vi "Fetch.vi"(6 "Prune Branches?":bool, 8 "error in (no error)":errorcluster, 10 "Name/Remote URL":string, 11 "Git Implementation in":refnum<class "Git Implementation.lvclass">) -> (0 "error out":errorcluster, 2 "Status Message":string, 3 "Git Implementation out":refnum<class "Git Implementation.lvclass">)   [LabVIEW 2017, in "Git-LabVIEW.lvlib" / "Git Implementation.lvclass"]
doc: "Fetches (updates) a repository from the remote by name or URL.\nWhen no name is specified, the default remote will be used (this is often called \"origin\").\nDo not use the Status Message as a parseable output - it is for user information/display only and may change between versions."
uses:
  Git Implementation.lvclass
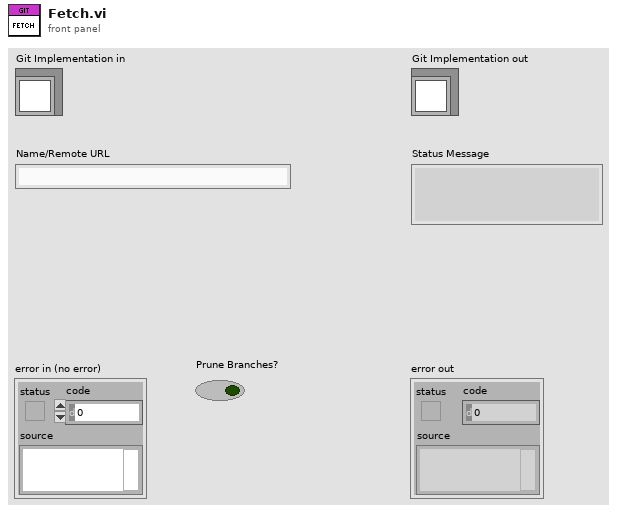
[diagram p1: front panel]
types:
  T1 = typedef "Git-LabVIEW.lvlib/Git Implementation.lvclass/CMD Return.ctl" = cluster{"StdOut":string, "StdErr":string, "Return Code":i32}
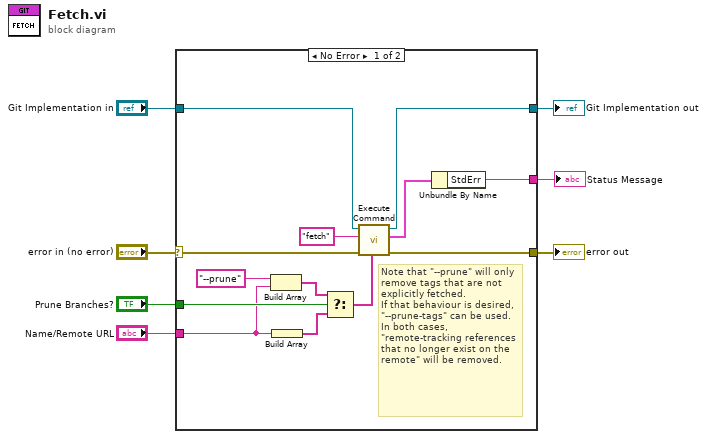
[diagram p0: block diagram]
diagram:
  n1 = case shown="No Error" "error in (no error)" {
    selector: "error in (no error)" -> [w20 w22]
    tunnel: [w15 w22] -> w6
    tunnel: [w18 w21] -> w4
    tunnel: "Git Implementation in" -> [w19 w21]
    tunnel: "Name/Remote URL" -> [w10 _]
    tunnel: [w14 _] -> w2
    tunnel: "Prune Branches?" -> [w13 _]
    frame No Error {
      # "Note that \"--prune\" will only remove tags that are not explicitly fetched.\nIf that behaviour is desired, \"--prune-tags\" can be used.\nIn both cases, \"remote-tracking references that no longer exist on the remote\" will be removed."
      n2 = Build Array("--prune" ("element"), w10) -> (w8:string[])
      n3 = Build Array(w10) -> (w12:string[])
      n4 = Select(t=w8, s=w13, f=w12) -> (s? t:f=w11:string[])
      n5 = call "Execute Command.vi"("Arguments"=w11, "error in (no error)"=w20, "Command"="fetch", "Git Implementation in"=w19) -> ("error out"=w15:errorcluster, "CMD Return"=w16:T1, "Git Implementation out"=w18:refnum<class "Git Implementation.lvclass">)  [unwired: 5 in]
      n6 = Unbundle By Name(w16) -> ("StdErr"=w14:string)
    }
    frame Error {
    }
  }
  "error out" <- w6
  "Git Implementation out" <- w4
  "Status Message" <- w2
